vi "Class to Variant.vi"(8 "error in (no error)":errorcluster, 11 "Build Job in":refnum<class "Build Job.lvclass">) -> (0 "error out":errorcluster, 1 "Display":string, 2 "Data":variant, 3 "Build Job out":refnum<class "Build Job.lvclass">)   [LabVIEW 2014, in "Build Job.lvclass"]
uses:
  Build Job.lvclass
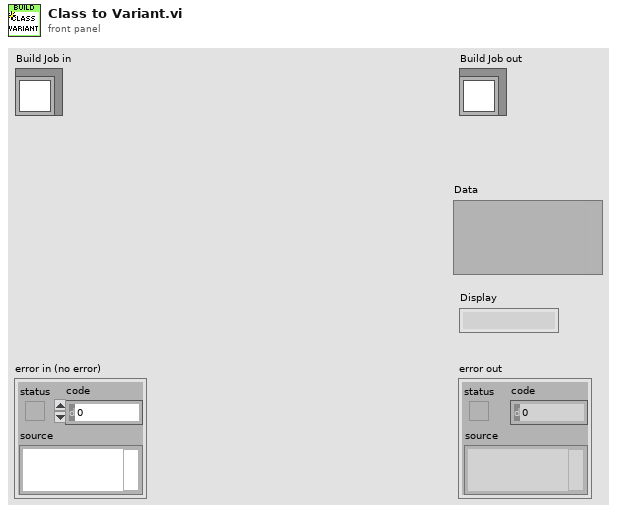
[diagram p1: front panel]
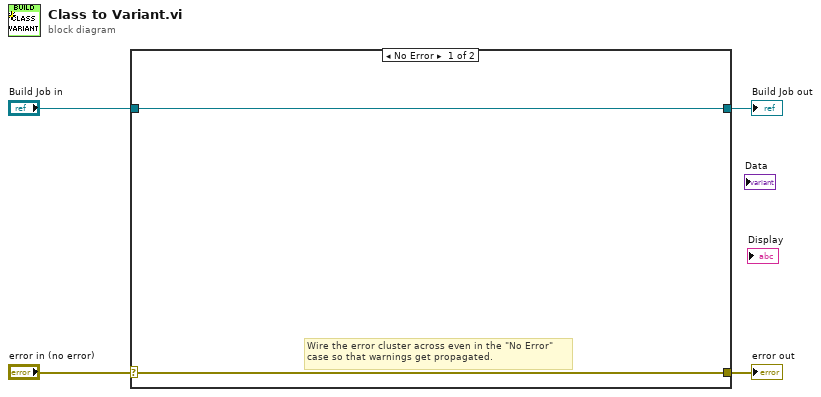
[diagram p0: block diagram]
diagram:
  n1 = case shown="No Error" "error in (no error)" {
    selector: "error in (no error)" -> [w5 w8]
    tunnel: [w5 w8] -> w3
    tunnel: [w6 w7] -> w1
    tunnel: "Build Job in" -> [w6 w7]
    frame No Error {
      # "Wire the error cluster across even in the \"No Error\"\ncase so that warnings get propagated."
    }
    frame Error {
    }
  }
  "error out" <- w3
  "Build Job out" <- w1
